vi "All object detection ver2.vi"(0 "Image In":T2, 1 "error in":errorcluster) -> (2 "Image Out":T2, 3 "Object detection count":T1, 4 "error out":errorcluster)   [LabVIEW 2018]
uses:
  <vilib>/vision/Image Controls.llb/IMAQ Image.ctl
panel:
  out "Shape Report (calibrated) (Locate hair gel)":T3(array[cluster]) {"Score" format="%.2f"; "Centroid"."y" format="%.2f"; "Centroid"."x" format="%.2f"}
  out "Matches (calibrated) (Locate red ball)":T4(array[cluster]) {"Bounding Box"."y" format="%.2f"; "Bounding Box"."x" format="%.2f"; "Position"."y" format="%.2f"; "Position"."x" format="%.2f"; "Score" format="%.2f"; "Scale" format="%.2f"; "Angle" format="%.2f"}
  out "Shape Report (calibrated) (Locate pipe)":T3(array[cluster]) {"Score" format="%.2f"; "Centroid"."y" format="%.2f"; "Centroid"."x" format="%.2f"}
  out "Shape Report (calibrated) (Locate soap)":T3(array[cluster]) {"Score" format="%.2f"; "Centroid"."y" format="%.2f"; "Centroid"."x" format="%.2f"}
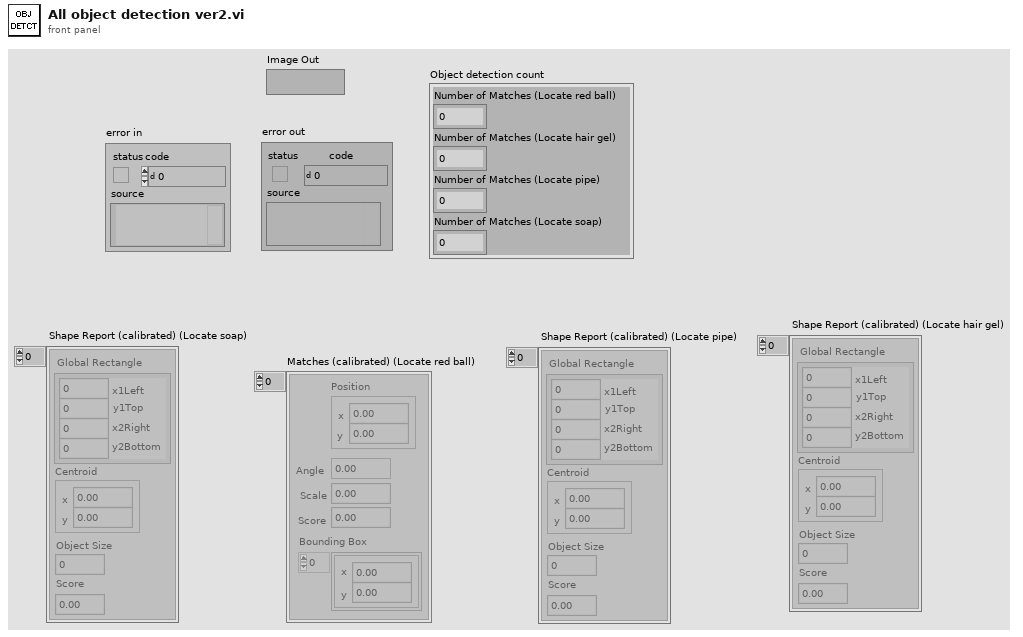
[diagram p1: front panel]
types:
  T1 = cluster{"Number of Matches (Locate red ball)":i32, "Number of Matches (Locate hair gel)":i32, "Number of Matches (Locate pipe)":i32, "Number of Matches (Locate soap)":i32}
  T2 = typedef "IMAQ Image.ctl" = refnum<image>
  T3 = cluster{"Global Rectangle":cluster{"x1Left":i32, "y1Top":i32, "x2Right":i32, "y2Bottom":i32}, "Centroid":cluster{"x":sgl, "y":sgl}, "Object Size":u32, "Score":dbl}[]
  T4 = cluster{"Position":cluster{"x":sgl, "y":sgl}, "Angle":sgl, "Scale":sgl, "Score":sgl, "Bounding Box":cluster{"x":sgl, "y":sgl}[]}[]
  T5 = cluster{"Shape Report (calibrated) (Locate soap)[0]":cluster{"Global Rectangle":cluster{"x1Left":i32, "y1Top":i32, "x2Right":i32, "y2Bottom":i32}, "Centroid":cluster{"x":sgl, "y":sgl}, "Object Size":u32, "Score":dbl}, "Shape Report (calibrated) (Locate soap)[1]":cluster{"Global Rectangle":cluster{"x1Left":i32, "y1Top":i32, "x2Right":i32, "y2Bottom":i32}, "Centroid":cluster{"x":sgl, "y":sgl}, "Object Size":u32, "Score":dbl}, "Shape Report (calibrated) (Locate soap)[2]":cluster{"Global Rectangle":cluster{"x1Left":i32, "y1Top":i32, "x2Right":i32, "y2Bottom":i32}, "Centroid":cluster{"x":sgl, "y":sgl}, "Object Size":u32, "Score":dbl}, "Shape Report (calibrated) (Locate soap)[3]":cluster{"Global Rectangle":cluster{"x1Left":i32, "y1Top":i32, "x2Right":i32, "y2Bottom":i32}, "Centroid":cluster{"x":sgl, "y":sgl}, "Object Size":u32, "Score":dbl}, "Shape Report (calibrated) (Locate soap)[4]":cluster{"Global Rectangle":cluster{"x1Left":i32, "y1Top":i32, "x2Right":i32, "y2Bottom":i32}, "Centroid":cluster{"x":sgl, "y":sgl}, "Object Size":u32, "Score":dbl}, "Shape Report (calibrated) (Locate soap)[5]":cluster{"Global Rectangle":cluster{"x1Left":i32, "y1Top":i32, "x2Right":i32, "y2Bottom":i32}, "Centroid":cluster{"x":sgl, "y":sgl}, "Object Size":u32, "Score":dbl}, "Shape Report (calibrated) (Locate soap)[6]":cluster{"Global Rectangle":cluster{"x1Left":i32, "y1Top":i32, "x2Right":i32, "y2Bottom":i32}, "Centroid":cluster{"x":sgl, "y":sgl}, "Object Size":u32, "Score":dbl}, "Shape Report (calibrated) (Locate soap)[7]":cluster{"Global Rectangle":cluster{"x1Left":i32, "y1Top":i32, "x2Right":i32, "y2Bottom":i32}, "Centroid":cluster{"x":sgl, "y":sgl}, "Object Size":u32, "Score":dbl}, "Shape Report (calibrated) (Locate soap)[8]":cluster{"Global Rectangle":cluster{"x1Left":i32, "y1Top":i32, "x2Right":i32, "y2Bottom":i32}, "Centroid":cluster{"x":sgl, "y":sgl}, "Object Size":u32, "Score":dbl}}
  T6 = cluster{"Shape Report (calibrated) (Locate hair gel)[0]":cluster{"Global Rectangle":cluster{"x1Left":i32, "y1Top":i32, "x2Right":i32, "y2Bottom":i32}, "Centroid":cluster{"x":sgl, "y":sgl}, "Object Size":u32, "Score":dbl}, "Shape Report (calibrated) (Locate hair gel)[1]":cluster{"Global Rectangle":cluster{"x1Left":i32, "y1Top":i32, "x2Right":i32, "y2Bottom":i32}, "Centroid":cluster{"x":sgl, "y":sgl}, "Object Size":u32, "Score":dbl}, "Shape Report (calibrated) (Locate hair gel)[2]":cluster{"Global Rectangle":cluster{"x1Left":i32, "y1Top":i32, "x2Right":i32, "y2Bottom":i32}, "Centroid":cluster{"x":sgl, "y":sgl}, "Object Size":u32, "Score":dbl}, "Shape Report (calibrated) (Locate hair gel)[3]":cluster{"Global Rectangle":cluster{"x1Left":i32, "y1Top":i32, "x2Right":i32, "y2Bottom":i32}, "Centroid":cluster{"x":sgl, "y":sgl}, "Object Size":u32, "Score":dbl}, "Shape Report (calibrated) (Locate hair gel)[4]":cluster{"Global Rectangle":cluster{"x1Left":i32, "y1Top":i32, "x2Right":i32, "y2Bottom":i32}, "Centroid":cluster{"x":sgl, "y":sgl}, "Object Size":u32, "Score":dbl}, "Shape Report (calibrated) (Locate hair gel)[5]":cluster{"Global Rectangle":cluster{"x1Left":i32, "y1Top":i32, "x2Right":i32, "y2Bottom":i32}, "Centroid":cluster{"x":sgl, "y":sgl}, "Object Size":u32, "Score":dbl}, "Shape Report (calibrated) (Locate hair gel)[6]":cluster{"Global Rectangle":cluster{"x1Left":i32, "y1Top":i32, "x2Right":i32, "y2Bottom":i32}, "Centroid":cluster{"x":sgl, "y":sgl}, "Object Size":u32, "Score":dbl}, "Shape Report (calibrated) (Locate hair gel)[7]":cluster{"Global Rectangle":cluster{"x1Left":i32, "y1Top":i32, "x2Right":i32, "y2Bottom":i32}, "Centroid":cluster{"x":sgl, "y":sgl}, "Object Size":u32, "Score":dbl}, "Shape Report (calibrated) (Locate hair gel)[8]":cluster{"Global Rectangle":cluster{"x1Left":i32, "y1Top":i32, "x2Right":i32, "y2Bottom":i32}, "Centroid":cluster{"x":sgl, "y":sgl}, "Object Size":u32, "Score":dbl}}
  T7 = cluster{"Shape Report (calibrated) (Locate pipe)[0]":cluster{"Global Rectangle":cluster{"x1Left":i32, "y1Top":i32, "x2Right":i32, "y2Bottom":i32}, "Centroid":cluster{"x":sgl, "y":sgl}, "Object Size":u32, "Score":dbl}, "Shape Report (calibrated) (Locate pipe)[1]":cluster{"Global Rectangle":cluster{"x1Left":i32, "y1Top":i32, "x2Right":i32, "y2Bottom":i32}, "Centroid":cluster{"x":sgl, "y":sgl}, "Object Size":u32, "Score":dbl}, "Shape Report (calibrated) (Locate pipe)[2]":cluster{"Global Rectangle":cluster{"x1Left":i32, "y1Top":i32, "x2Right":i32, "y2Bottom":i32}, "Centroid":cluster{"x":sgl, "y":sgl}, "Object Size":u32, "Score":dbl}, "Shape Report (calibrated) (Locate pipe)[3]":cluster{"Global Rectangle":cluster{"x1Left":i32, "y1Top":i32, "x2Right":i32, "y2Bottom":i32}, "Centroid":cluster{"x":sgl, "y":sgl}, "Object Size":u32, "Score":dbl}, "Shape Report (calibrated) (Locate pipe)[4]":cluster{"Global Rectangle":cluster{"x1Left":i32, "y1Top":i32, "x2Right":i32, "y2Bottom":i32}, "Centroid":cluster{"x":sgl, "y":sgl}, "Object Size":u32, "Score":dbl}, "Shape Report (calibrated) (Locate pipe)[5]":cluster{"Global Rectangle":cluster{"x1Left":i32, "y1Top":i32, "x2Right":i32, "y2Bottom":i32}, "Centroid":cluster{"x":sgl, "y":sgl}, "Object Size":u32, "Score":dbl}, "Shape Report (calibrated) (Locate pipe)[6]":cluster{"Global Rectangle":cluster{"x1Left":i32, "y1Top":i32, "x2Right":i32, "y2Bottom":i32}, "Centroid":cluster{"x":sgl, "y":sgl}, "Object Size":u32, "Score":dbl}, "Shape Report (calibrated) (Locate pipe)[7]":cluster{"Global Rectangle":cluster{"x1Left":i32, "y1Top":i32, "x2Right":i32, "y2Bottom":i32}, "Centroid":cluster{"x":sgl, "y":sgl}, "Object Size":u32, "Score":dbl}, "Shape Report (calibrated) (Locate pipe)[8]":cluster{"Global Rectangle":cluster{"x1Left":i32, "y1Top":i32, "x2Right":i32, "y2Bottom":i32}, "Centroid":cluster{"x":sgl, "y":sgl}, "Object Size":u32, "Score":dbl}}
  T8 = cluster{"Matches (calibrated) (Locate red ball)[0]":cluster{"Position":cluster{"x":sgl, "y":sgl}, "Angle":sgl, "Scale":sgl, "Score":sgl, "Bounding Box":cluster{"x":sgl, "y":sgl}[]}, "Matches (calibrated) (Locate red ball)[1]":cluster{"Position":cluster{"x":sgl, "y":sgl}, "Angle":sgl, "Scale":sgl, "Score":sgl, "Bounding Box":cluster{"x":sgl, "y":sgl}[]}, "Matches (calibrated) (Locate red ball)[2]":cluster{"Position":cluster{"x":sgl, "y":sgl}, "Angle":sgl, "Scale":sgl, "Score":sgl, "Bounding Box":cluster{"x":sgl, "y":sgl}[]}, "Matches (calibrated) (Locate red ball)[3]":cluster{"Position":cluster{"x":sgl, "y":sgl}, "Angle":sgl, "Scale":sgl, "Score":sgl, "Bounding Box":cluster{"x":sgl, "y":sgl}[]}, "Matches (calibrated) (Locate red ball)[4]":cluster{"Position":cluster{"x":sgl, "y":sgl}, "Angle":sgl, "Scale":sgl, "Score":sgl, "Bounding Box":cluster{"x":sgl, "y":sgl}[]}, "Matches (calibrated) (Locate red ball)[5]":cluster{"Position":cluster{"x":sgl, "y":sgl}, "Angle":sgl, "Scale":sgl, "Score":sgl, "Bounding Box":cluster{"x":sgl, "y":sgl}[]}, "Matches (calibrated) (Locate red ball)[6]":cluster{"Position":cluster{"x":sgl, "y":sgl}, "Angle":sgl, "Scale":sgl, "Score":sgl, "Bounding Box":cluster{"x":sgl, "y":sgl}[]}, "Matches (calibrated) (Locate red ball)[7]":cluster{"Position":cluster{"x":sgl, "y":sgl}, "Angle":sgl, "Scale":sgl, "Score":sgl, "Bounding Box":cluster{"x":sgl, "y":sgl}[]}, "Matches (calibrated) (Locate red ball)[8]":cluster{"Position":cluster{"x":sgl, "y":sgl}, "Angle":sgl, "Scale":sgl, "Score":sgl, "Bounding Box":cluster{"x":sgl, "y":sgl}[]}}
  T9 = cluster{"Global Rectangle":cluster{"x1Left":i32, "y1Top":i32, "x2Right":i32, "y2Bottom":i32}, "Centroid":cluster{"x":sgl, "y":sgl}, "Object Size":u32, "Score":dbl}
  T10 = cluster{"Position":cluster{"x":sgl, "y":sgl}, "Angle":sgl, "Scale":sgl, "Score":sgl, "Bounding Box":cluster{"x":sgl, "y":sgl}[]}
  T11 = cluster{"x1Left":i32, "y1Top":i32, "x2Right":i32, "y2Bottom":i32}
  T12 = cluster{"Bounding Box[0]":cluster{"x":sgl, "y":sgl}, "Bounding Box[1]":cluster{"x":sgl, "y":sgl}, "Bounding Box[2]":cluster{"x":sgl, "y":sgl}, "Bounding Box[3]":cluster{"x":sgl, "y":sgl}, "Bounding Box[4]":cluster{"x":sgl, "y":sgl}, "Bounding Box[5]":cluster{"x":sgl, "y":sgl}, "Bounding Box[6]":cluster{"x":sgl, "y":sgl}, "Bounding Box[7]":cluster{"x":sgl, "y":sgl}, "Bounding Box[8]":cluster{"x":sgl, "y":sgl}}
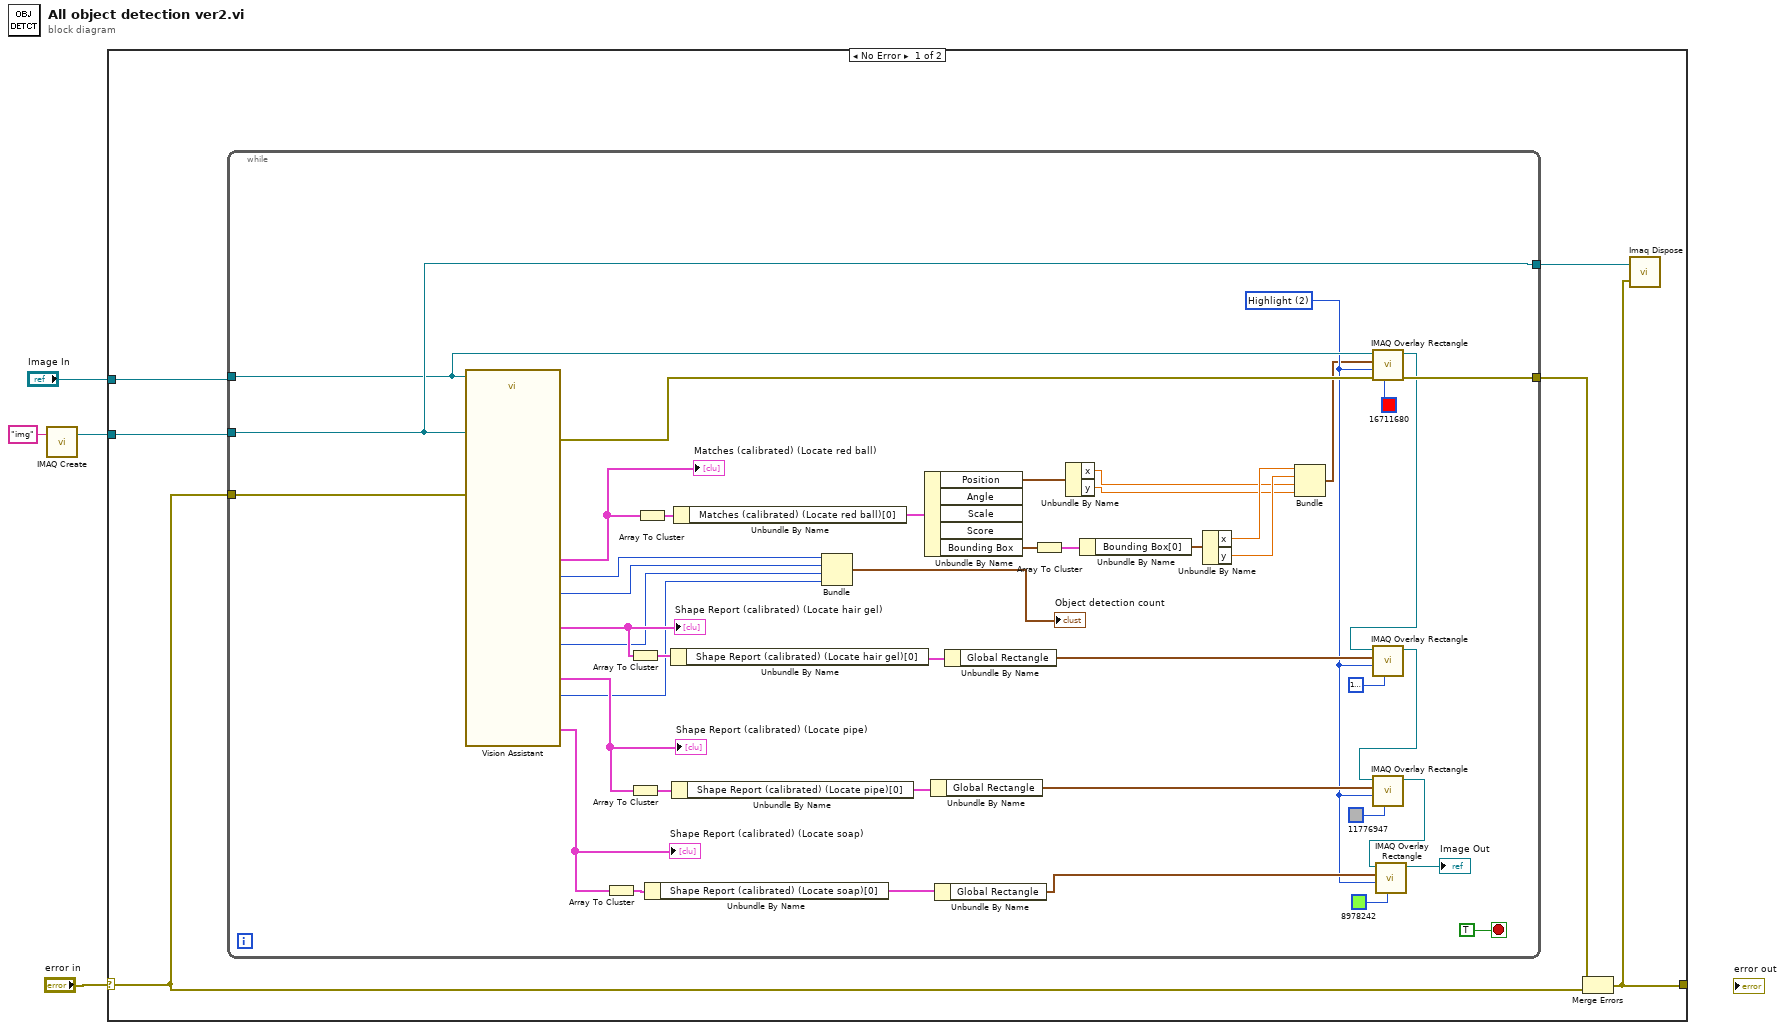
[diagram p0: block diagram]
diagram:
  n1 = call "IMAQ Create"("Image Name"="img") -> ("New Image"=w2:T2)  [unwired: 4 in, 1 out]
  n2 = case shown="No Error" "error in" {
    selector: "error in" -> [w10 w55]
    tunnel: [w8 w55] -> _
    tunnel: w2 -> [w6 _]
    tunnel: "Image In" -> [w5 _]
    frame No Error {
      n3 = while {
        tunnel: w10 -> [w17]
        tunnel: w6 -> [w40]
        tunnel: [w40] -> w9
        tunnel: [w38] -> w7
        tunnel: w5 -> [w37]
        stop <- TRUE stop-if-true
        w30 = u32 2 items=["Frame", "Fill", "Highlight"] ("Drawing Mode (Frame)")
        n4 = call "Vision Assistant"("Image In"=w37, "Image Dst"=w40, "error in"=w17) -> ("Shape Report (calibrated) (Locate soap)"=w29:T3, "Number of Matches (Locate soap)"=w12:i32, "Shape Report (calibrated) (Locate pipe)"=w43:T3, "Number of Matches (Locate pipe)"=w13:i32, "Matches (calibrated) (Locate red ball)"=w48:T4, "Number of Matches (Locate red ball)"=w15:i32, "Number of Matches (Locate hair gel)"=w14:i32, "Shape Report (calibrated) (Locate hair gel)"=w45:T3, "error out"=w39:errorcluster)  [unwired: 11 in, 5 out]
        "Shape Report (calibrated) (Locate soap)" <- w29
        "Shape Report (calibrated) (Locate pipe)" <- w43
        "Matches (calibrated) (Locate red ball)" <- w48
        "Shape Report (calibrated) (Locate hair gel)" <- w45
        n5 = Array To Cluster(array=w29) -> (cluster=w23:T5)
        n6 = Array To Cluster(array=w45) -> (cluster=w46:T6)
        n7 = Array To Cluster(array=w43) -> (cluster=w42:T7)
        n8 = Array To Cluster(array=w48) -> (cluster=w53:T8)
        n9 = Unbundle By Name(w23) -> ("Shape Report (calibrated) (Locate soap)[0]"=w28:T9)
        n10 = Unbundle By Name(w46) -> ("Shape Report (calibrated) (Locate hair gel)[0]"=w44:T9)
        n11 = Unbundle By Name(w42) -> ("Shape Report (calibrated) (Locate pipe)[0]"=w41:T9)
        n12 = Unbundle By Name(w53) -> ("Matches (calibrated) (Locate red ball)[0]"=w47:T10)
        n13 = Bundle("Number of Matches (Locate red ball)"=w15, "Number of Matches (Locate hair gel)"=w14, "Number of Matches (Locate pipe)"=w13, "Number of Matches (Locate soap)"=w12) -> (→"Object detection count":T1)  [unwired: 1 in]
        n14 = Unbundle By Name(w47) -> ("Position"=w49:cluster{"x":sgl, "y":sgl}, "Bounding Box"=w52:cluster{"x":sgl, "y":sgl}[])  [unwired: 3 out]
        n15 = Unbundle By Name(w41) -> ("Global Rectangle"=w34:T11)
        n16 = Unbundle By Name(w28) -> ("Global Rectangle"=w31:T11)
        n17 = Unbundle By Name(w44) -> ("Global Rectangle"=w35:T11)
        n18 = Array To Cluster(array=w52) -> (cluster=w51:T12)
        n19 = Unbundle By Name(w49) -> ("x"=w20:sgl, "y"=w19:sgl)
        n20 = Unbundle By Name(w51) -> ("Bounding Box[0]"=w50:cluster{"x":sgl, "y":sgl})
        n21 = Unbundle By Name(w50) -> ("x"=w22:sgl, "y"=w21:sgl)
        n22 = Bundle("x"=w22, "y"=w21, "x"=w20, "y"=w19) -> (w18:cluster{"x":sgl, "y":sgl, "x":sgl, "y":sgl})  [unwired: 1 in]
        n23 = call "IMAQ Overlay Rectangle"("Color"=u32 16711680, "error in (no error)"=w39, "Drawing Mode (Frame)"=w30, "Rectangle"=w18, "Image"=w37) -> ("error out"=w38:errorcluster, "Image Out"=w36:T2)  [unwired: 5 in]
        n24 = call "IMAQ Overlay Rectangle"("Color"=u32 16777226, "Drawing Mode (Frame)"=w30, "Rectangle"=w35, "Image"=w36) -> ("Image Out"=w33:T2)  [unwired: 6 in, 1 out]
        n25 = call "IMAQ Overlay Rectangle"("Color"=u32 11776947, "Drawing Mode (Frame)"=w30, "Rectangle"=w34, "Image"=w33) -> ("Image Out"=w32:T2)  [unwired: 6 in, 1 out]
        n26 = call "IMAQ Overlay Rectangle"("Color"=u32 8978242, "Drawing Mode (Frame)"=w30, "Rectangle"=w31, "Image"=w32) -> ("Image Out"=→"Image Out":T2)  [unwired: 6 in, 1 out]
      }
      n27 = Merge Errors(w7, w10) -> (w8:errorcluster)
      n28 = call "Imaq Dispose"("Image"=w9, "error in (no error)"=w8) -> ()  [unwired: 4 in, 1 out]
    }
    frame Error {
    }
  }
